vi "Func-엑셀 데이터를 그래프로 출력.vi"() -> ()   [LabVIEW 2015] (continued)
\n85\t85\t89.708\n85\t85\t89.71\n85\t85\t89.709\n85\t85\t89.709\n85\t85\t89.711\n85\t85\t89.717\n85\t85\t89.716\n85\t85\t89.715\n85\t85\t89.719\n85\t85\t89.72\n85\t85\t89.723\n85\t85\t89.722\n85\t85\t89.725\n85\t85\t89.726\n85\t85\t89.723\n85\t85\t89.725\n85\t85\t89.723\n85\t85\t89.728\n85\t85\t89.728\n85\t85\t89.731\n85\t85\t89.733\n85\t85\t89.734\n85\t85\t89.736\n85\t85\t89.734\n85\t85\t89.727\n85\t85\t89.725\n85\t85\t89.724\n85\t85\t89.724\n85\t85\t89.723\n85\t85\t89.723\n85\t85\t89.727\n85\t85\t89.728\n85\t85\t89.727\n85\t85\t89.723\n85\t85\t89.721\n85\t85\t89.719\n85\t85\t89.718\n85\t85\t89.719\n85\t85\t89.72\n85\t85\t89.725\n85\t85\t89.724\n85\t85\t89.725\n85\t85\t89.727\n85\t85\t89.726\n85\t85\t89.727\n85\t85\t89.725\n85\t85\t89.729\n85\t85\t89.725\n85\t85\t89.723\n85\t85\t89.721\n85\t85\t89.721\n85\t85\t89.721\n85\t85\t89.721\n85\t85\t89.722\n85\t85\t89.727\n85\t85\t89.727\n85\t85\t89.729\n85\t85\t89.73\n85\t85\t89.734\n85\t85\t89.732\n85\t85\t89.727\n85\t85\t89.73\n85\t85\t89.728\n85\t85\t89.731\n85\t85\t89.729\n85\t85\t89.728\n85\t85\t89.73\n85\t85\t89.732\n85\t85\t89.738\n85\t85\t89.733\n85\t85\t89.733\n85\t85\t89.736\n85\t85\t89.736\n85\t85\t89.737\n85\t85\t89.731\n85\t85\t89.733\n85\t85\t89.734\n85\t85\t89.732\n85\t85\t89.732\n85\t85\t89.729\n85\t85\t89.732\n85\t85\t89.732\n85\t85\t89.734\n85\t85\t89.731\n85\t85\t89.733\n85\t85\t89.735\n85\t85\t89.736\n85\t85\t89.735\n85\t85\t89.732\n85\t85\t89.735\n85\t85\t89.733\n85\t85\t89.735\n85\t85\t89.73\n85\t85\t89.73\n85\t85\t89.729\n85\t85\t89.729\n85\t85\t89.733\n85\t85\t89.729\n85\t85\t89.731\n85\t85\t89.732\n85\t85\t89.734\n85\t85\t89.734\n85\t85\t89.732\n85\t85\t89.734\n85\t85\t89.736\n85\t85\t89.743\n85\t85\t89.745\n85\t85\t89.744\n85\t85\t89.741\n85\t85\t89.741\n85\t85\t89.742\n85\t85\t89.738\n85\t85\t89.736\n85\t85\t89.738\n85\t85\t89.743\n85\t85\t89.74\n85\t85\t89.739\n85\t85\t89.738\n85\t85\t89.739\n85\t85\t89.738\n85\t85\t89.738\n85\t85\t89.742\n85\t85\t89.742\n85\t85\t89.745\n85\t85\t89.738\n85\t85\t89.74\n85\t85\t89.734\n85\t85\t89.734\n85\t85\t89.736\n85\t85\t89.73\n85\t85\t89.735\n85\t85\t89.732\n85\t85\t89.736\n85\t85\t89.735\n85\t85\t89.736\n85\t85\t89.74\n85\t85\t89.739\n85\t85\t89.744\n85\t85\t89.741\n85\t85\t89.739\n85\t85\t89.738\n85\t85\t89.743\n85\t85\t89.742\n85\t85\t89.737\n85\t85\t89.74\n85\t85\t89.744\n85\t85\t89.744\n85\t85\t89.742\n85\t85\t89.743\n85\t85\t89.744\n85\t85\t89.742\n85\t85\t89.743\n85\t85\t89.745\n85\t85\t89.741\n85\t85\t89.735\n85\t85\t89.737\n85\t85\t89.741\n85\t85\t89.737\n85\t85\t89.736\n85\t85\t89.739\n85\t85\t89.746\n85\t85\t89.745\n85\t85\t89.742\n85\t85\t89.743\n85\t85\t89.741\n85\t85\t89.743\n85\t85\t89.741\n85\t85\t89.741\n85\t85\t89.739\n85\t85\t89.743\n85\t85\t89.743\n85\t85\t89.745\n85\t85\t89.745\n85\t85\t89.746\n85\t85\t89.752\n85\t85\t89.751\n85\t85\t89.751\n85\t85\t89.751\n85\t85\t89.747\n85\t85\t89.743\n85\t85\t89.74\n85\t85\t89.738\n85\t85\t89.741\n85\t85\t89.738\n85\t85\t89.745\n85\t85\t89.745\n85\t85\t89.743\n85\t85\t89.745\n85\t85\t89.744\n85\t85\t89.745\n85\t85\t89.745\n85\t85\t89.746\n85\t85\t89.746\n85\t85\t89.744\n85\t85\t89.743\n85\t85\t89.744\n85\t85\t89.739\n85\t85\t89.742\n85\t85\t89.746\n85\t85\t89.747\n85\t85\t89.752\n85\t85\t89.752\n85\t85\t89.756\n85\t85\t89.755\n85\t85\t89.751\n85\t85\t89.753\n85\t85\t89.752\n85\t85\t89.749\n85\t85\t89.749\n85\t85\t89.754\n85\t85\t89.755\n85\t85\t89.752\n85\t85\t89.745\n85\t85\t89.751\n85\t85\t89.749\n85\t85\t89.746\n85\t85\t89.745\n85\t85\t89.746\n85\t85\t89.75\n85\t85\t89.749\n85\t85\t89.749\n85\t85\t89.748\n85\t85\t89.748\n85\t85\t89.75\n85\t85\t89.749\n85\t85\t89.751\n85\t85\t89.751\n85\t85\t89.751\n85\t85\t89.75\n85\t85\t89.748\n85\t85\t89.75\n85\t85\t89.75\n85\t85\t89.751\n85\t85\t89.75\n85\t85\t89.754\n85\t85\t89.754\n85\t85\t89.754\n85\t85\t89.752\n85\t85\t89.749\n85\t85\t89.753\n85\t85\t89.752\n85\t85\t89.751\n85\t85\t89.748\n85\t85\t89.75\n85\t85\t89.754\n85\t85\t89.755\n85\t85\t89.755\n85\t85\t89.758\n85\t85\t89.76\n85\t85\t89.764\n85\t85\t89.762\n85\t85\t89.76\n85\t85\t89.757\n85\t85\t89.756\n85\t85\t89.754\n85\t85\t89.749\n85\t85\t89.752\n85\t85\t89.753\n85\t85\t89.755\n85\t85\t89.752\n85\t85\t89.75\n85\t85\t89.755\n85\t85\t89.755\n85\t85\t89.757\n85\t85\t89.758\n85\t85\t89.758\n85\t85\t89.759\n85\t85\t89.761\n85\t85\t89.759\n85\t85\t89.757\n85\t85\t89.756\n85\t85\t89.757\n85\t85\t89.755\n85\t85\t89.755\n85\t85\t89.752\n85\t85\t89.753\n85\t85\t89.756\n85\t85\t89.756\n85\t85\t89.758\n85\t85\t89.757\n85\t85\t89.759\n85\t85\t89.759\n85\t85\t89.754\n85\t85\t89.754\n85\t85\t89.757\n85\t85\t89.759\n85\t85\t89.76\n85\t85\t89.759\n85\t85\t89.761\n85\t85\t89.764\n85\t85\t89.761\n85\t85\t89.758\n85\t85\t89.757\n85\t85\t89.759\n85\t85\t89.757\n85\t85\t89.756\n85\t85\t89.757\n85\t85\t89.759\n85\t85\t89.758\n85\t85\t89.76\n85\t85\t89.758\n85\t85\t89.761\n85\t85\t89.759\n85\t85\t89.764\n85\t85\t89.761\n85\t85\t89.759\n85\t85\t89.76\n85\t85\t89.757\n85\t85\t89.756\n85\t85\t89.756\n85\t85\t89.759\n85\t85\t89.757\n85\t85\t89.759\n85\t85\t89.76\n85\t85\t89.764\n85\t85\t89.758\n85\t85\t89.758\n85\t85\t89.759\n85\t85\t89.756\n85\t85\t89.756\n85\t85\t89.757\n85\t85\t89.76\n85\t85\t89.761\n85\t85\t89.764\n85\t85\t89.769\n85\t85\t89.768\n85\t85\t89.766\n85\t85\t89.759\n85\t85\t89.757\n85\t85\t89.757\n85\t85\t89.757\n85\t85\t89.756\n85\t85\t89.757\n85\t85\t89.76\n85\t85\t89.762\n85\t85\t89.763\n85\t85\t89.766\n85\t85\t89.767\n85\t85\t89.766\n85\t85\t89.768\n85\t85\t89.765\n85\t85\t89.759\n85\t85\t89.761\n85\t85\t89.761\n85\t85\t89.764\n85\t85\t89.767\n85\t85\t89.77\n85\t85\t89.77\n85\t85\t89.768\n85\t85\t89.768\n85\t85\t89.763\n85\t85\t89.761\n85\t85\t89.759\n85\t85\t89.759\n85\t85\t89.759\n85\t85\t89.757\n85\t85\t89.761\n85\t85\t89.759\n85\t85\t89.757\n85\t85\t89.756\n85\t85\t89.757\n85\t85\t89.759\n85\t85\t89.76\n85\t85\t89.763\n85\t85\t89.767\n85\t85\t89.767\n85\t85\t89.762\n85\t85\t89.761\n85\t85\t89.76\n85\t85\t89.761\n85\t85\t89.759\n85\t85\t89.761\n85\t85\t89.764\n85\t85\t89.767\n85\t85\t89.769\n85\t85\t89.766\n85\t85\t89.771\n85\t85\t89.772\n85\t85\t89.77\n85\t85\t89.77\n85\t85\t89.764\n85\t85\t89.764\n85\t85\t89.76\n85\t85\t89.762\n85\t85\t89.761\n85\t85\t89.761\n85\t85\t89.764\n85\t85\t89.762\n85\t85\t89.759\n85\t85\t89.754\n85\t85\t89.755\n85\t85\t89.754\n85\t85\t89.756\n85\t85\t89.757\n85\t85\t89.762\n85\t85\t89.767\n85\t85\t89.769\n85\t85\t89.768\n85\t85\t89.772\n85\t85\t89.775\n85\t85\t89.774\n85\t85\t89.776\n85\t85\t89.777\n85\t85\t89.777\n85\t85\t89.778\n85\t85\t89.777\n85\t85\t89.773\n85\t85\t89.771\n85\t85\t89.771\n85\t85\t89.774\n85\t85\t89.767\n85\t85\t89.766\n85\t85\t89.771\n84.917\t84.93\t89.842\n84.833\t84.87\t89.835\n84.75\t84.97\t89.841\n84.667\t84.9\t89.837\n84.583\t84.79\t89.839\n84.5\t84.65\t89.844\n84.417\t84.48\t89.846\n84.333\t84.29\t89.846\n84.25\t84.09\t89.839\n84.167\t83.86\t89.844\n84.083\t83.63\t89.843\n84\t83.4\t89.845\n83.917\t83.18\t89.843\n83.833\t82.97\t89.847\n83.75\t82.77\t89.841\n83.667\t82.59\t89.84\n83.583\t82.42\t89.832\n83.5\t82.27\t89.822\n83.417\t82.14\t89.823\n83.333\t82.01\t89.814\n83.25\t81.91\t89.816\n83.167\t81.82\t89.802\n83.083\t81.74\t89.791\n83\t81.68\t89.791\n82.917\t81.62\t89.779\n82.833\t81.56\t89.764\n82.75\t81.52\t89.752\n82.667\t81.46\t89.737\n82.583\t81.41\t89.732\n82.5\t81.35\t89.716\n82.417\t81.31\t89.709\n82.333\t81.24\t89.695\n82.25\t81.18\t89.68\n82.167\t81.11\t89.654\n82.083\t81.04\t89.648\n82\t80.98\t89.615\n81.917\t80.91\t89.611\n81.833\t80.85\t89.583\n81.75\t80.77\t89.565\n81.667\t80.7\t89.539\n81.583\t80.62\t89.518\n81.5\t80.54\t89.492\n81.417\t80.45\t89.482\n81.333\t80.37\t89.451\n81.25\t80.29\t89.428\n81.167\t80.19\t89.405\n81.083\t80.12\t89.375\n81\t80.02\t89.353\n80.917\t79.93\t89.333\n80.833\t79.84\t89.312\n80.75\t79.76\t89.272\n80.667\t79.66\t89.242\n80.583\t79.57\t89.216\n80.5\t79.48\t89.19\n80.417\t79.39\t89.16\n80.333\t79.3\t89.128\n80.25\t79.22\t89.098\n80.167\t79.14\t89.063\n80.083\t79.06\t89.044\n80\t78.97\t89.001\n79.917\t78.9\t88.966\n79.833\t78.82\t88.939\n79.75\t78.73\t88.906\n79.667\t78.64\t88.866\n79.583\t78.56\t88.834\n79.5\t78.48\t88.8\n79.417\t78.4\t88.76\n79.333\t78.31\t88.727\n79.25\t78.23\t88.69\n79.167\t78.14\t88.65\n79.083\t78.06\t88.623\n79\t77.97\t88.575\n78.917\t77.89\t88.532\n78.833\t77.8\t88.504\n78.75\t77.73\t88.458\n78.667\t77.65\t88.422\n78.583\t77.56\t88.376\n78.5\t77.48\t88.334\n78.417\t77.41\t88.298\n78.333\t77.33\t88.26\n78.25\t77.25\t88.209\n78.167\t77.17\t88.169\n78.083\t77.09\t88.127\n78\t77.02\t88.084\n77.917\t76.94\t88.036\n77.833\t76.86\t87.988\n77.75\t76.79\t87.953\n77.667\t76.71\t87.896\n77.583\t76.62\t87.863\n77.5\t76.54\t87.807\n77.417\t76.47\t87.776\n77.333\t76.39\t87.725\n77.25\t76.3\t87.674\n77.167\t76.22\t87.625\n77.083\t76.15\t87.577\n77\t76.07\t87.539\n76.917\t75.98\t87.475\n76.833\t75.89\t87.44\n76.75\t75.8\t87.368\n76.667\t75.72\t87.338\n76.583\t75.64\t87.268\n76.5\t75.55\t87.228\n76.417\t75.47\t87.177\n76.333\t75.39\t87.125\n76.25\t75.32\t87.084\n76.167\t75.24\t87.021\n76.083\t75.17\t86.976\n76\t75.09\t86.927\n75.917\t75.02\t86.867\n75.833\t74.92\t86.815\n75.75\t74.85\t86.765\n75.667\t74.76\t86.711\n75.583\t74.68\t86.655\n75.5\t74.59\t86.609\n75.417\t74.5\t86.553\n75.333\t74.41\t86.493\n75.25\t74.33\t86.433\n75.167\t74.25\t86.383\n75.083\t74.16\t86.332\n75\t74.08\t86.28\n74.917\t73.99\t86.217\n74.833\t73.91\t86.157\n74.75\t73.83\t86.103\n74.667\t73.74\t86.049\n74.583\t73.66\t85.989\n74.5\t73.57\t85.932\n74.417\t73.49\t85.872\n74.333\t73.41\t85.825\n74.25\t73.34\t85.763\n74.167\t73.25\t85.709\n74.083\t73.18\t85.649\n74\t73.1\t85.593\n73.917\t73.02\t85.532\n73.833\t72.93\t85.482\n73.75\t72.84\t85.412\n73.667\t72.76\t85.342\n73.583\t72.68\t85.297\n73.5\t72.59\t85.239\n73.417\t72.51\t85.164\n73.333\t72.42\t85.108\n73.25\t72.34\t85.054\n73.167\t72.26\t84.992\n73.083\t72.19\t84.93\n73\t72.1\t84.874\n72.917\t72.02\t84.809\n72.833\t71.93\t84.745\n72.75\t71.85\t84.686\n72.667\t71.77\t84.619\n72.583\t71.68\t84.553\n72.5\t71.6\t84.502\n72.417\t71.52\t84.436\n72.333\t71.45\t84.378\n72.25\t71.37\t84.325\n72.167\t71.29\t84.245\n72.083\t71.22\t84.189\n72\t71.13\t84.123\n71.917\t71.05\t84.056\n71.833\t70.97\t83.996\n71.75\t70.88\t83.929\n71.667\t70.81\t83.862\n71.583\t70.71\t83.804\n71.5\t70.63\t83.747\n71.417\t70.54\t83.675\n71.333\t70.45\t83.609\n71.25\t70.37\t83.547\n71.167\t70.3\t83.479\n71.083\t70.22\t83.411\n71\t70.12\t83.342\n70.917\t70.05\t83.287\n70.833\t69.97\t83.223\n70.75\t69.9\t83.152\n70.667\t69.81\t83.082\n70.583\t69.73\t83.021\n70.5\t69.66\t82.954\n70.417\t69.57\t82.887\n70.333\t69.5\t82.815\n70.25\t69.4\t82.753\n70.167\t69.33\t82.691\n70.083\t69.25\t82.621\n70\t69.17\t82.546\n69.917\t69.09\t82.485\n69.833\t68.99\t82.42\n69.75\t68.91\t82.349\n69.667\t68.83\t82.286\n69.583\t68.75\t82.221\n69.5\t68.67\t82.155\n69.417\t68.58\t82.086\n69.333\t68.5\t82.016\n69.25\t68.41\t81.947\n69.167\t68.33\t81.878\n69.083\t68.25\t81.808\n69\t68.16\t81.738\n68.917\t68.09\t81.663\n68.833\t68.02\t81.602\n68.75\t67.95\t81.538\n68.667\t67.86\t81.461\n68.583\t67.79\t81.389\n68.5\t67.71\t81.321\n68.417\t67.63\t81.261\n68.333\t67.55\t81.19\n68.25\t67.46\t81.122\n68.167\t67.38\t81.049\n68.083\t67.31\t80.972\n68\t67.23\t80.904\n67.917\t67.15\t80.836\n67.833\t67.08\t80.765\n67.75\t66.99\t80.693\n67.667\t66.91\t80.627\n67.583\t66.82\t80.555\n67.5\t66.73\t80.482\n67.417\t66.66\t80.418\n67.333\t66.57\t80.348\n67.25\t66.49\t80.271\n67.167\t66.42\t80.201\n67.083\t66.33\t80.134\n67\t66.25\t80.059\n66.917\t66.18\t79.99\n66.833\t66.09\t79.916\n66.75\t66.01\t79.855\n66.667\t65.91\t79.782\n66.583\t65.83\t79.71\n66.5\t65.75\t79.638\n66.417\t65.67\t79.562\n66.333\t65.58\t79.49\n66.25\t65.49\t79.421\n66.167\t65.4\t79.355\n66.083\t65.32\t79.284\n66\t65.24\t79.209\n65.917\t65.17\t79.137\n65.833\t65.08\t79.066\n65.75\t64.99\t78.995\n65.667\t64.92\t78.919\n65.583\t64.83\t78.834\n65.5\t64.75\t78.772\n65.417\t64.67\t78.702\n65.333\t64.59\t78.634\n65.25\t64.5\t78.564\n65.167\t64.42\t78.488\n65.083\t64.33\t78.41\n65\t64.24\t78.347\n64.917\t64.16\t78.27\n65\t64.08\t78.201\n65\t64.08\t78.192\n65\t64.07\t78.187\n65\t64.06\t78.181\n65\t64.05\t78.173\n65\t64.04\t78.164\n65\t64.03\t78.154\n65\t64.02\t78.149\n65\t64.01\t78.139\n65\t64\t78.127\n65\t63.99\t78.115\n65\t63.98\t78.106\n65\t63.98\t78.101\n65\t63.97\t78.093\n65\t63.96\t78.087\n65\t63.95\t78.086\n65\t63.94\t78.084\n65\t63.93\t78.073\n65\t63.92\t78.069\n65\t63.92\t78.061\n65\t63.91\t78.05\n65\t63.9\t78.039\n65\t63.89\t78.031\n65\t63.88\t78.025\n65\t63.87\t78.018\n65\t63.87\t78.013\n65\t63.87\t78.005\n65\t63.86\t78.002\n65\t63.85\t77.997\n65\t63.84\t77.988\n65\t63.84\t77.979\n65\t63.83\t77.971\n65\t63.83\t77.967\n65\t63.82\t77.956\n65\t63.81\t77.947\n65\t63.81\t77.937\n65\t63.8\t77.933\n65\t63.79\t77.928\n65\t63.79\t77.922\n65\t63.78\t77.918\n65\t63.78\t77.907\n65\t63.77\t77.902\n65\t63.77\t77.897\n65\t63.77\t77.887\n65\t63.77\t77.877\n65\t63.77\t77.868\n65\t63.76\t77.864\n65\t63.76\t77.859\n65\t63.75\t77.842\n65\t63.75\t77.834\n65\t63.75\t77.83\n65\t63.74\t77.821\n65\t63.74\t77.815\n65\t63.74\t77.809\n65\t63.73\t77.8\n65\t63.73\t77.797\n65\t63.73\t77.788\n65\t63.73\t77.781\n65\t63.73\t77.772\n65\t63.73\t77.767\n65\t63.73\t77.761\n65\t63.72\t77.751\n65\t63.72\t77.745\n65\t63.72\t77.734\n65\t63.72\t77.73\n65\t63.71\t77.722\n65\t63.71\t77.716\n65\t63.71\t77.708\n65\t63.71\t77.705\n65\t63.71\t77.7\n65\t63.71\t77.691\n65\t63.71\t77.681\n65\t63.71\t77.673\n65\t63.71\t77.669\n65\t63.71\t77.659\n65\t63.71\t77.651\n65\t63.71\t77.648\n65\t63.71\t77.638\n65\t63.71\t77.629\n65\t63.71\t77.62\n65\t63.71\t77.613\n65\t63.71\t77.606\n65\t63.72\t77.597\n65\t63.72\t77.59\n65\t63.72\t77.585\n65\t63.73\t77.58\n65\t63.73\t77.573\n65\t63.73\t77.566\n65\t63.73\t77.557\n65\t63.73\t77.552\n65\t63.74\t77.544\n65\t63.74\t77.534\n65\t63.74\t77.524\n65\t63.74\t77.519\n65\t63.74\t77.505\n65\t63.75\t77.499\n65\t63.75\t77.494\n65\t63.75\t77.489\n65\t63.75\t77.483\n65\t63.76\t77.473\n65\t63.76\t77.469\n65\t63.76\t77.458\n65\t63.76\t77.451\n65\t63.77\t77.438\n65\t63.77\t77.432\n65\t63.77\t77.429\n65\t63.77\t77.422\n65\t63.77\t77.418\n65\t63.77\t77.412\n65\t63.78\t77.404\n65\t63.78\t77.401\n65\t63.79\t77.39\n65\t63.8\t77.38\n65\t63.8\t77.374\n65\t63.81\t77.365\n65\t63.81\t77.365\n65\t63.81\t77.354\n65\t63.81\t77.35\n65\t63.82\t77.346\n65\t63.82\t77.338\n65\t63.83\t77.329\n65\t63.83\t77.32\n65\t63.84\t77.314\n65\t63.84\t77.3\n65\t63.85\t77.29\n65\t63.85\t77.282\n65\t63.85\t77.273\n65\t63.86\t77.263\n65\t63.86\t77.258\n65\t63.87\t77.253\n65\t63.87\t77.245\n65\t63.87\t77.234\n65\t63.87\t77.23\n65\t63.88\t77.227\n65\t63.88\t77.221\n65\t63.89\t77.213\n65\t63.9\t77.206\n65\t63.9\t77.202\n65\t63.91\t77.193\n65\t63.91\t77.186\n65\t63.92\t77.176\n65\t63.92\t77.17\n65\t63.93\t77.166\n65\t63.93\t77.155\n65\t63.94\t77.153\n65\t63.94\t77.139\n65\t63.95\t77.133\n65\t63.96\t77.125\n65\t63.96\t77.116\n65\t63.97\t77.107\n65\t63.97\t77.096\n65\t63.98\t77.093\n65\t63.98\t77.086\n65\t63.98\t77.082\n65\t63.99\t77.07\n65\t64\t77.067\n65\t64\t77.062\n65\t64\t77.051\n65\t64.01\t77.043\n65\t64.02\t77.034\n65\t64.02\t77.027\n65\t64.03\t77.019\n65\t64.04\t77.008\n65\t64.04\t77.008\n65\t64.05\t77.005\n65\t64.05\t76.998\n65\t64.05\t76.992\n65\t64.06\t76.988\n65\t64.07\t76.982\n65\t64.07\t76.975\n65\t64.08\t76.966\n65\t64.08\t76.955\n65\t64.08\t76.951\n65\t64.09\t76.945\n65\t64.09\t76.941\n65\t64.1\t76.933\n65\t64.1\t76.927\n65\t64.11\t76.921\n65\t64.11\t76.911\n65\t64.12\t76.898\n65\t64.13\t76.886\n65\t64.13\t76.88\n65\t64.14\t76.873\n65\t64.14\t76.866\n65\t64.15\t76.859\n65\t64.15\t76.855\n65\t64.16\t76.85\n65\t64.16\t76.843\n65\t64.16\t76.831\n65\t64.17\t76.827\n65\t64.17\t76.823\n65\t64.18\t76.811\n65\t64.18\t76.807\n65\t64.18\t76.8\n65\t64.19\t76.791\n65\t64.19\t76.787\n65\t64.2\t76.78\n65\t64.2\t76.774\n65\t64.21\t76.765\n65\t64.22\t76.755\n65\t64.22\t76.753\n65\t64.23\t76.744\n65\t64.23\t76.734\n65\t64.23\t76.729\n65\t64.24\t76.725\n65\t64.24\t76.716\n65\t64.25\t76.708\n65\t64.25\t76.702\n65\t64.26\t76.695\n65\t64.26\t76.688\n65\t64.27\t76.68\n65\t64.28\t76.671\n65\t64.28\t76.664\n65\t64.28\t76.659\n65\t64.28\t76.655\n65\t64.29\t76.647\n65\t64.29\t76.64\n65\t64.29\t76.636\n65\t64.3\t76.63\n65\t64.3\t76.617\n65\t64.31\t76.61\n65\t64.31\t76.607\n65\t64.32\t76.598\n65\t64.33\t76.589\n65\t64.33\t76.582\n65\t64.34\t76.573\n65\t64.34\t76.567\n65\t64.35\t76.56\n65\t64.35\t76.55\n65\t64.36\t76.543\n65\t64.37\t76.536\n65\t64.37\t76.533\n65\t64.37\t76.524\n65\t64.38\t76.517\n65\t64.38\t76.515\n65\t64.38\t76.513\n65\t64.38\t76.505\n65\t64.38\t76.498\n65\t64.39\t76.491\n65\t64.39\t76.482\n65\t64.4\t76.471\n65\t64.41\t76.463\n65\t64.41\t76.454\n65\t64.41\t76.446\n65\t64.41\t76.44\n65\t64.42\t76.429\n65\t64.42\t76.425\n65\t64.43\t76.418\n65\t64.43\t76.412\n65\t64.44\t76.408\n65\t64.44\t76.402\n65\t64.45\t76.399\n65\t64.45\t76.392\n65\t64.46\t76.386\n65\t64.47\t76.381\n65\t64.47\t76.371\n65\t64.47\t76.361\n65\t64.48\t76.355\n65\t64.48\t76.35\n65\t64.48\t76.343\n65\t64.48\t76.331\n65\t64.49\t76.328\n65\t64.49\t76.319\n65\t64.5\t76.314\n65\t64.5\t76.306\n65\t64.51\t76.296\n65\t64.51\t76.291\n65\t64.51\t76.286\n65\t64.51\t76.277\n65\t64.52\t76.272\n65\t64.52\t76.271\n65\t64.53\t76.265\n65\t64.53\t76.258\n65\t64.53\t76.252\n65\t64.53\t76.249\n65\t64.54\t76.239\n65\t64.54\t76.23\n65\t64.54\t76.223\n65\t64.55\t76.218\n65\t64.55\t76.206\n65\t64.56\t76.198\n65\t64.56\t76.195\n65\t64.56\t76.186\n65\t64.57\t76.18\n65\t64.57\t76.175\n65\t64.57\t76.169\n65\t64.58\t76.163\n65\t64.58\t76.157\n65\t64.59\t76.148\n65\t64.59\t76.14\n65\t64.59\t76.135\n65\t64.59\t76.125\n65\t64.59\t76.12\n65\t64.6\t76.111\n65\t64.6\t76.104\n65\t64.61\t76.098\n65\t64.61\t76.087\n65\t64.61\t76.084\n65\t64.61\t76.077\n65\t64.61\t76.074\n65\t64.62\t76.07\n65\t64.62\t76.068\n65\t64.62\t76.062\n65\t64.62\t76.054\n65\t64.63\t76.045\n65\t64.63\t76.03\n65\t64.63\t76.023\n65\t64.64\t76.014\n65\t64.64\t76.006\n65\t64.64\t76.002\n65\t64.64\t76\n65\t64.65\t75.997\n65\t64.65\t75.991\n65\t64.65\t75.983\n65\t64.65\t75.977\n65\t64.66\t75.971\n65\t64.66\t75.963\n65\t64.66\t75.951\n65\t64.66\t75.949\n65\t64.67\t75.943\n65\t64.67\t75.939\n65\t64.67\t75.932\n65\t64.67\t75.927\n65\t64.68\t75.922\n65\t64.68\t75.911\n65\t64.69\t75.906\n65\t64.69\t75.898\n65\t64.69\t75.896\n65\t64.69\t75.887\n65\t64.69\t75.884\n65\t64.69\t75.882\n65\t64.69\t75.871\n65\t64.69\t75.867\n65\t64.69\t75.859\n65\t64.69\t75.854\n65\t64.7\t75.845\n65\t64.7\t75.838\n65\t64.7\t75.832\n65\t64.71\t75.825\n65\t64.71\t75.821\n65\t64.72\t75.815\n65\t64.72\t75.811\n65\t64.72\t75.804\n65\t64.73\t75.796\n65\t64.73\t75.791\n65\t64.73\t75.779\n65\t64.73\t75.773\n65\t64.73\t75.77\n65\t64.74\t75.762\n65\t64.74\t75.757\n65\t64.74\t75.755\n65\t64.74\t75.747\n65\t64.75\t75.741\n65\t64.75\t75.736\n65\t64.75\t75.73\n65\t64.75\t75.724\n65\t64.75\t75.715\n65\t64.75\t75.713\n65\t64.75\t75.709\n65\t64.76\t75.698\n65\t64.76\t75.689\n65\t64.76\t75.685\n65\t64.76\t75.68\n65\t64.76\t75.672\n65\t64.77\t75.667\n65\t64.76\t75.663\n65\t64.77\t75.658\n65\t64.77\t75.655\n65\t64.77\t75.646\n65\t64.77\t75.642\n65\t64.78\t75.637\n65\t64.78\t75.627\n65\t64.78\t75.621\n65\t64.78\t75.614\n65\t64.78\t75.608\n65\t64.79\t75.6\n65\t64.79\t75.593\n65\t64.79\t75.586\n65\t64.79\t75.583\n65\t64.79\t75.575\n65\t64.79\t75.576\n65\t64.79\t75.574\n65\t64.79\t75.565\n65\t64.8\t75.557\n65\t64.8\t75.551\n65\t64.8\t75.544\n65\t64.8\t75.534\n65\t64.8\t75.526\n65\t64.8\t75.523\n65\t64.8\t75.521\n65\t64.8\t75.516\n65\t64.8\t75.508\n65\t64.8\t75.505\n65\t64.8\t75.5\n65\t64.8\t75.49\n65\t64.81\t75.485\n65\t64.81\t75.484\n65\t64.81\t75.478\n65\t64.81\t75.471\n65\t64.82\t75.464\n65\t64.82\t75.461\n65\t64.82\t75.457\n65\t64.82\t75.444\n65\t64.82\t75.437\n65\t64.82\t75.432\n65\t64.82\t75.426\n65\t64.82\t75.418\n65\t64.82\t75.41\n65\t64.82\t75.405\n65\t64.82\t75.405\n65\t64.82\t75.396\n65\t64.82\t75.391\n65\t64.82\t75.389\n65\t64.82\t75.387\n65\t64.83\t75.377\n65\t64.83\t75.368\n65\t64.83\t75.361\n65\t64.84\t75.355\n65\t64.84\t75.351\n65\t64.84\t75.343\n65\t64.83\t75.342\n65\t64.83\t75.339\n65\t64.84\t75.334\n65\t64.84\t75.328\n65\t64.84\t75.318\n65\t64.84\t75.311\n65\t64.85\t75.3\n65\t64.86\t75.294\n65\t64.87\t75.287\n65\t64.88\t75.279\n65\t64.89\t75.279\n
